vi "Enqueue or Dequeue Array elements.vi"(4 "Stop Button":bool, 9 "ADD":bool, 10 "Delete":bool, 11 "Insert New element":dbl) -> (2 "Sum of Array Elements":dbl, 3 "Output array":dbl[](array[numeric]))   [LabVIEW 2020]
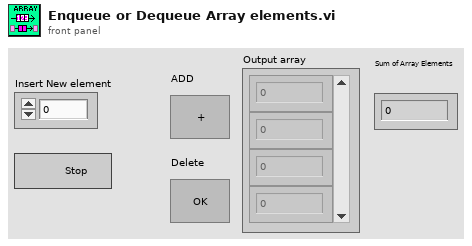
[diagram p1: front panel]
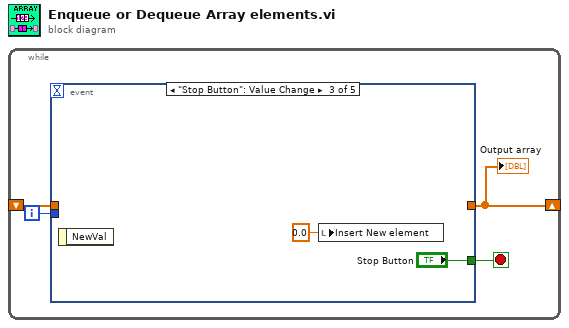
[diagram p0: block diagram]
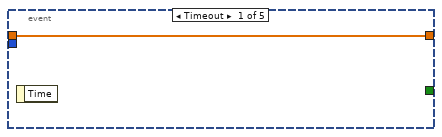
[diagram p2: hidden frame]
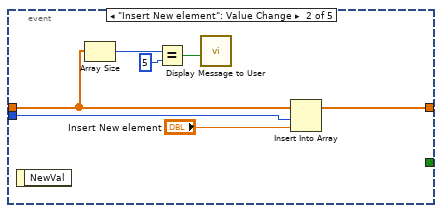
[diagram p3: hidden frame]
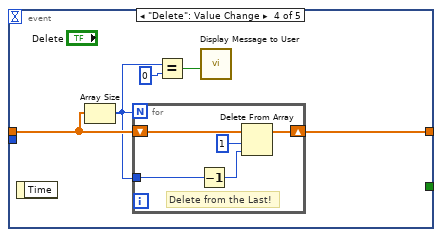
[diagram p4: hidden frame]
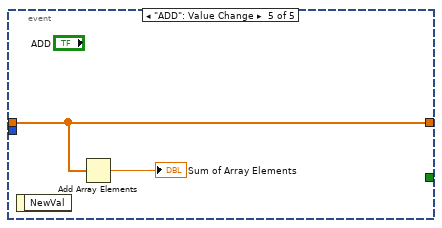
[diagram p5: hidden frame]
diagram:
  n1 = while {
    shift-right: [w3] -> _
    shift-left: _ -> [w4]
    i -> [w2]
    stop <- w1 stop-if-true
    n2 = event shown="[2] \"Stop Button\": Value Change" {
      selector: _ -> [_ _ _ _ _]
      dyn-events: _ -> [_ _ _ _ _]
      timeout: _ -> [_ _ _ _ _]
      tunnel: w4 -> [w5 w12 _ w19 w25]
      tunnel: [w5 w11 _ w18 w25] -> w3
      tunnel: w2 -> [_ w8 _ _ _]
      tunnel: [_ _ "Stop Button" _ _] -> w1
      event Timeout {
        n3 = event-data() -> ()  [unwired: 1 in, 1 out]
      }
      event "Insert New element": Value Change {
        n4 = event-data() -> ()  [unwired: 1 in, 1 out]
        n5 = Array Size(array=w12) -> (size(s)=w10:i32)
        n6 = Equal?(x=w10, y=5) -> (x = y?=w7:bool)
        n7 = call "Display Message to User"("Enable"=w7) -> ()  [unwired: 9 in, 2 out]
        n8 = Insert Into Array "Insert Into Array"(array=w12, index=w8, new element="Insert New element") -> (w11:dbl[])
      }
      event "Stop Button": Value Change {
        n9 = event-data() -> ()  [unwired: 1 in, 1 out]
        n10 = local write "Insert New element"(0.0 ("Insert New element")) -> ()
      }
      event "Delete": Value Change {
        n11 = event-data() -> ()  [unwired: 1 in, 1 out]
        n12 = Array Size(array=w19) -> (size(s)=w17:i32)
        n13 = for {
          N: w17 -> [_]
          shift-right: [w20] -> w18
          shift-left: w19 -> [w24]
          tunnel: w17 -> [w23]
          # "Delete from the Last!"
          n14 = Decrement(x=w23) -> (x-1=w22:i32)
          n15 = Delete From Array(array=w24, length=1, index=w22) -> (array with subset deleted=w20:dbl[])  [unwired: 1 out]
        }
        n16 = Equal?(x=w17, y=0) -> (x = y?=w15:bool)
        n17 = call "Display Message to User"("Enable"=w15) -> ()  [unwired: 9 in, 2 out]
      }
      event "ADD": Value Change {
        n18 = event-data() -> ()  [unwired: 1 in, 1 out]
        n19 = Add Array Elements(numeric array=w25) -> (sum=→"Sum of Array Elements":dbl)
      }
    }
    "Output array" <- w3
  }
